vi "Get Name.vi"(8 "error in":errorcluster, 11 "Material-Palette in":refnum<class "Material-Palette.lvclass">) -> (0 "error out":errorcluster, 2 "Name":string, 3 "Material-Palette out":refnum<class "Material-Palette.lvclass">)   [LabVIEW 2021, in "TSC Material Theme.lvlib" / "Material-Palette.lvclass"]
uses:
  Material-Palette.lvclass
  Material-Palette.lvclass/Material-Palette.ctl
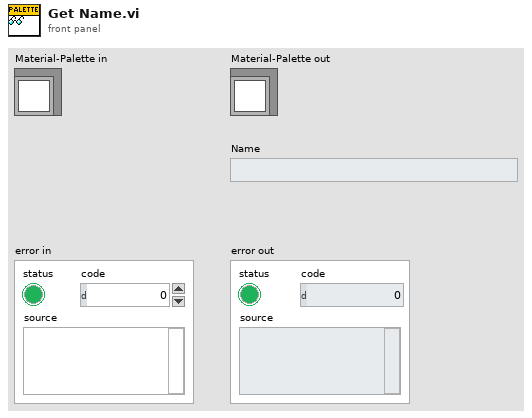
[diagram p1: front panel]
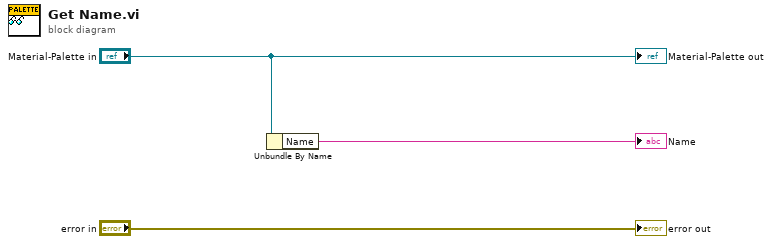
[diagram p0: block diagram]
diagram:
  n1 = Unbundle By Name("Material-Palette in") -> ("Name"=→"Name":string)
  "error out" <- "error in"
  "Material-Palette out" <- "Material-Palette in"
